vi "Open.vi"(8 "error in (no error)":errorcluster caption="entrée d'erreur (pas d'erreur)", 11 "Class Spectrum Analyser (Default) en entrée":refnum<class "Class Spectrum Analyser (Default).lvclass">) -> (0 "error out":errorcluster caption="sortie d'erreur", 3 "Class Spectrum Analyser (Default) en sortie":refnum<class "Class Spectrum Analyser (Default).lvclass">)   [LabVIEW 2020, in "Library Instrument & Equipement.lvlib" / "Library Spectrum Analyser.lvlib" / "Class Spectrum Analyser (Default).lvclass"]
uses:
  Class Spectrum Analyser (Default).lvclass
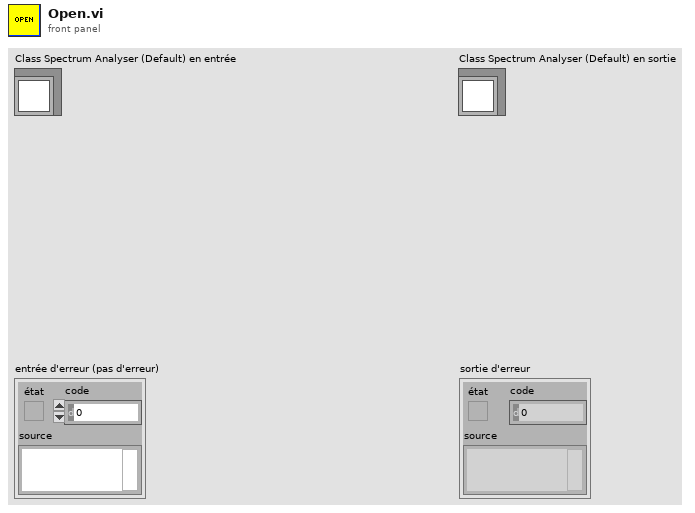
[diagram p1: front panel]
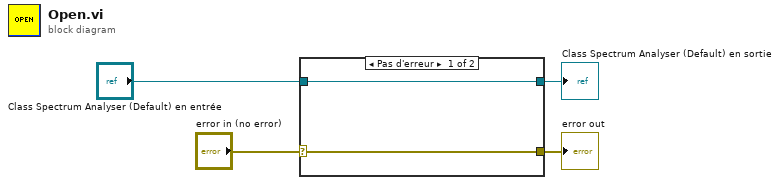
[diagram p0: block diagram]
diagram:
  n1 = case shown="Pas d'erreur" "error in (no error)" {
    selector: "error in (no error)" -> [w5 w8]
    tunnel: [w5 w8] -> w3
    tunnel: [w6 w7] -> w1
    tunnel: "Class Spectrum Analyser (Default) en entrée" -> [w6 w7]
    frame No Error {
    }
    frame Error {
    }
  }
  "error out" <- w3
  "Class Spectrum Analyser (Default) en sortie" <- w1
